vi "LJStreamUD.vi"() -> ()   [LabVIEW 2020]
uses:
  sub/LJstreamUD globals.vi
panel:
  out "Command Response  Error Message":string
  in  "Save Current Config":bool
  in  "Change Working Directory":bool
  in  "SettlingFactor":i32
  in  "Resolution":i32=1
  in  "Max File Size (Bytes)":i32=1048576 min=1 max=2000000000
  in  "Graph?":bool[](array[boolean])=[TRUE]
  out "Address":string
  in  "Disable Scaling*":bool=TRUE
  out "Device Type":string
  in  "stop stream":bool
  in  "exit":bool
  in  "# Scans On Graph":i32=1000 min=0
  out "Channel Config":T1={"# Channels"=4, "+Ch"=["0", "1", "2", "3", "4", "5", "6", "7"], "-Ch (U3)"=["31", "31", "31", "31", "31", "31", "31", "31"], "Ranges (UE9)"=[0, 0, 0, 0, 0, 0, 0, 0], "Scaling Equation"=["y=v0", "y=v1", "y=v2", "y=v3", "y=v4", "y=v5", "y=v6", "y=v7"]} {"Ranges (UE9)" items=["LJ_rgBIP5V", "LJ_rgUNI5V", "LJ_rgUNI2P5V", "LJ_rgUNI1P25V", "LJ_rgUNIP625V"]}
  out "Scaled":dbl[](array[numeric]) format="%.6f"
  in  "Scaling Equation":string[](array[string])=["y=a", "y=b", "y=c", "y=d", "y=e", "y=f", "y=g", "y=h", "y=i", "y=j", "y=k", "y=l", "y=m", "y=n", "y=o", "y=p"]
  in  "# Channels":i32=1 min=1
  in  "-Ch":string[](array[string])=["199", "199", "199", "199", "199", "199", "199", "199", "199", "199", "199", "199", "199", "199", "199", "199"]
  out "Voltage":dbl[](array[numeric]) format="%.6f"
  in  "Ranges":u16[](array[ring])=[0, 0, 0, 0, 0, 0, 0, 0, 0, 0, 0, 0, 0, 0, 0, 0] items=["LJ_rgBIP10V", "LJ_rgBIP5V", "LJ_rgUNI5V", "LJ_rgUNI2P5V", "LJ_rgUNI1P25V", "LJ_rgBIP1V", "LJ_rgUNIP625V", "LJ_rgBIPP1V", "LJ_rgBIPP01V"]
  out "?":cluster{dbl, dbl, dbl[][]}(graph)
  out "UD Backlog [%]":dbl format="%.2f"
  in  "+Ch":string[](array[string])=["0", "1", "2", "3", "4", "5", "6", "7", "8", "9", "10", "11", "12", "13", "14", "15"]
  out "ms Per Loop":u32
  out "Device Backlog [%]":dbl format="%.2f"
  out "# Scans Read":i32
  out "# of iterations":i32
  in  "Scan Rate (Hz)":dbl=500.0 format="%.3f"
  out "Current Data File":path
  in  "Data File Prefix":string="data"
  in  "Write To File":bool
  in  "start stream":bool caption="Start Stream"
  out "Last Stream Error Message":string
  # "0"
  # "1"
  # "2"
  # "3"
  # "4"
  # "5"
  # "6"
  # "7"
  # "8"
  # "9"
  # "10"
  # "11"
  # "12"
  # "13"
  # "14"
  # "15"
  # "*Scaling is computing intensive.  \nIf  the UD Backlog  is growing, disable scaling."
  # "# Iterations"
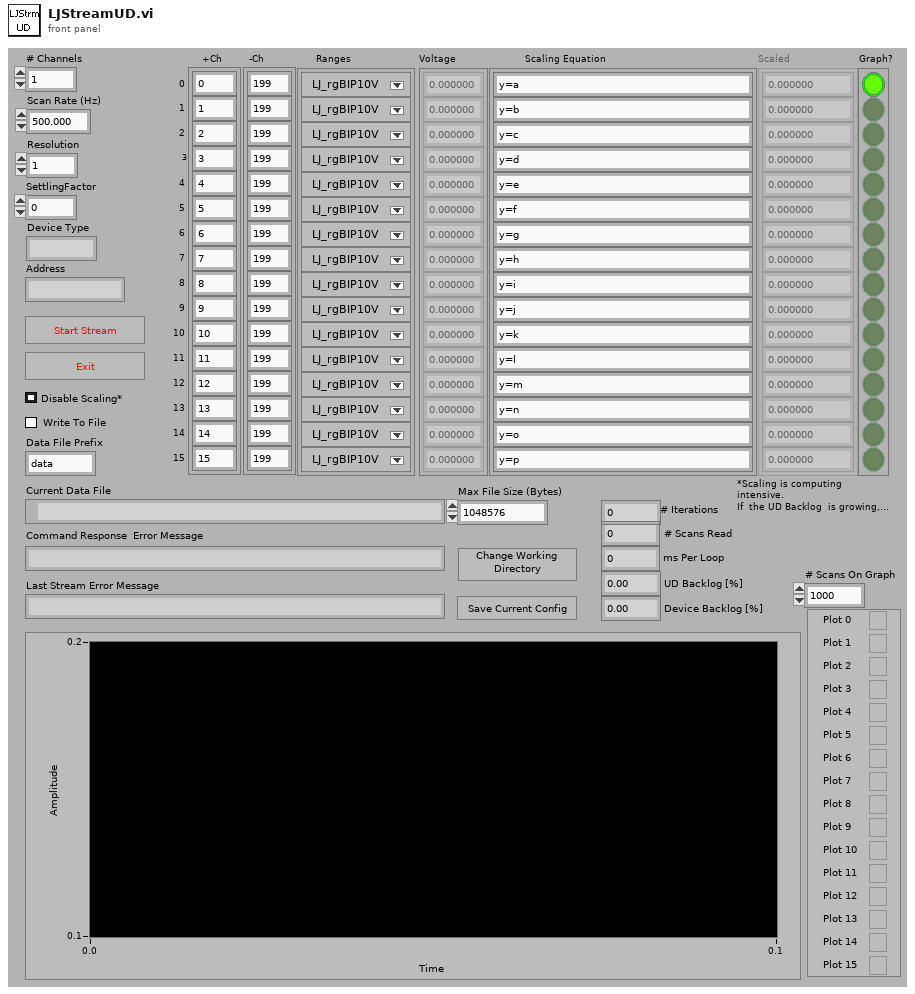
[diagram p1: front panel]
types:
  T1 = cluster{"# Channels":i32, "+Ch":string[], "-Ch (U3)":string[], "Ranges (UE9)":u16[], "Scaling Equation":string[]}
  T2 = cluster{"+Ch":string[], "-Ch":string[], "Ranges":u16[], "Scaling Equation":string[], "Graph?":bool[]}
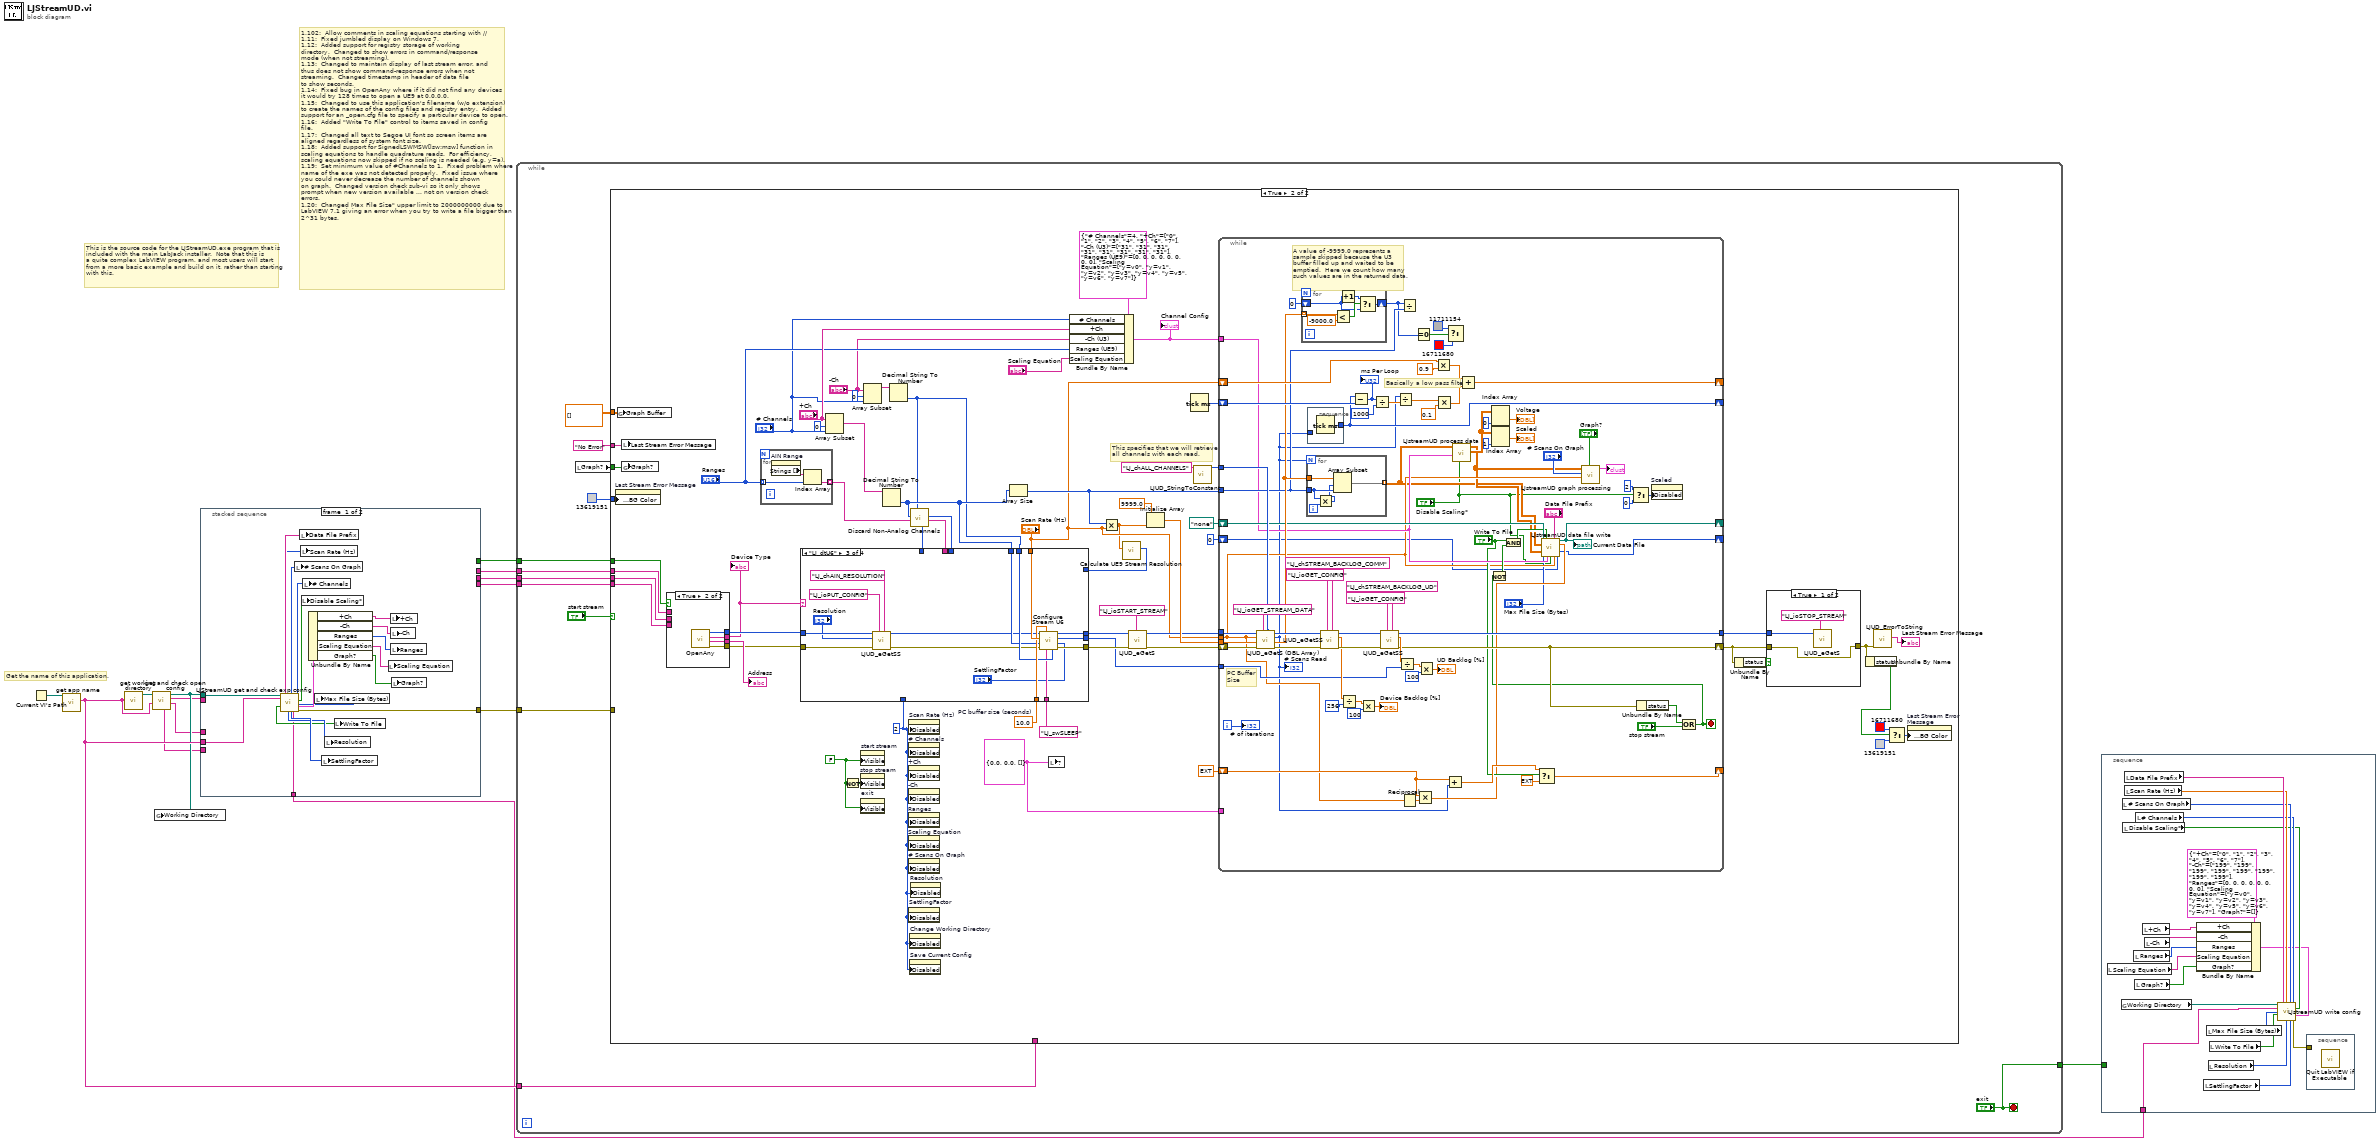
[diagram p0: block diagram]
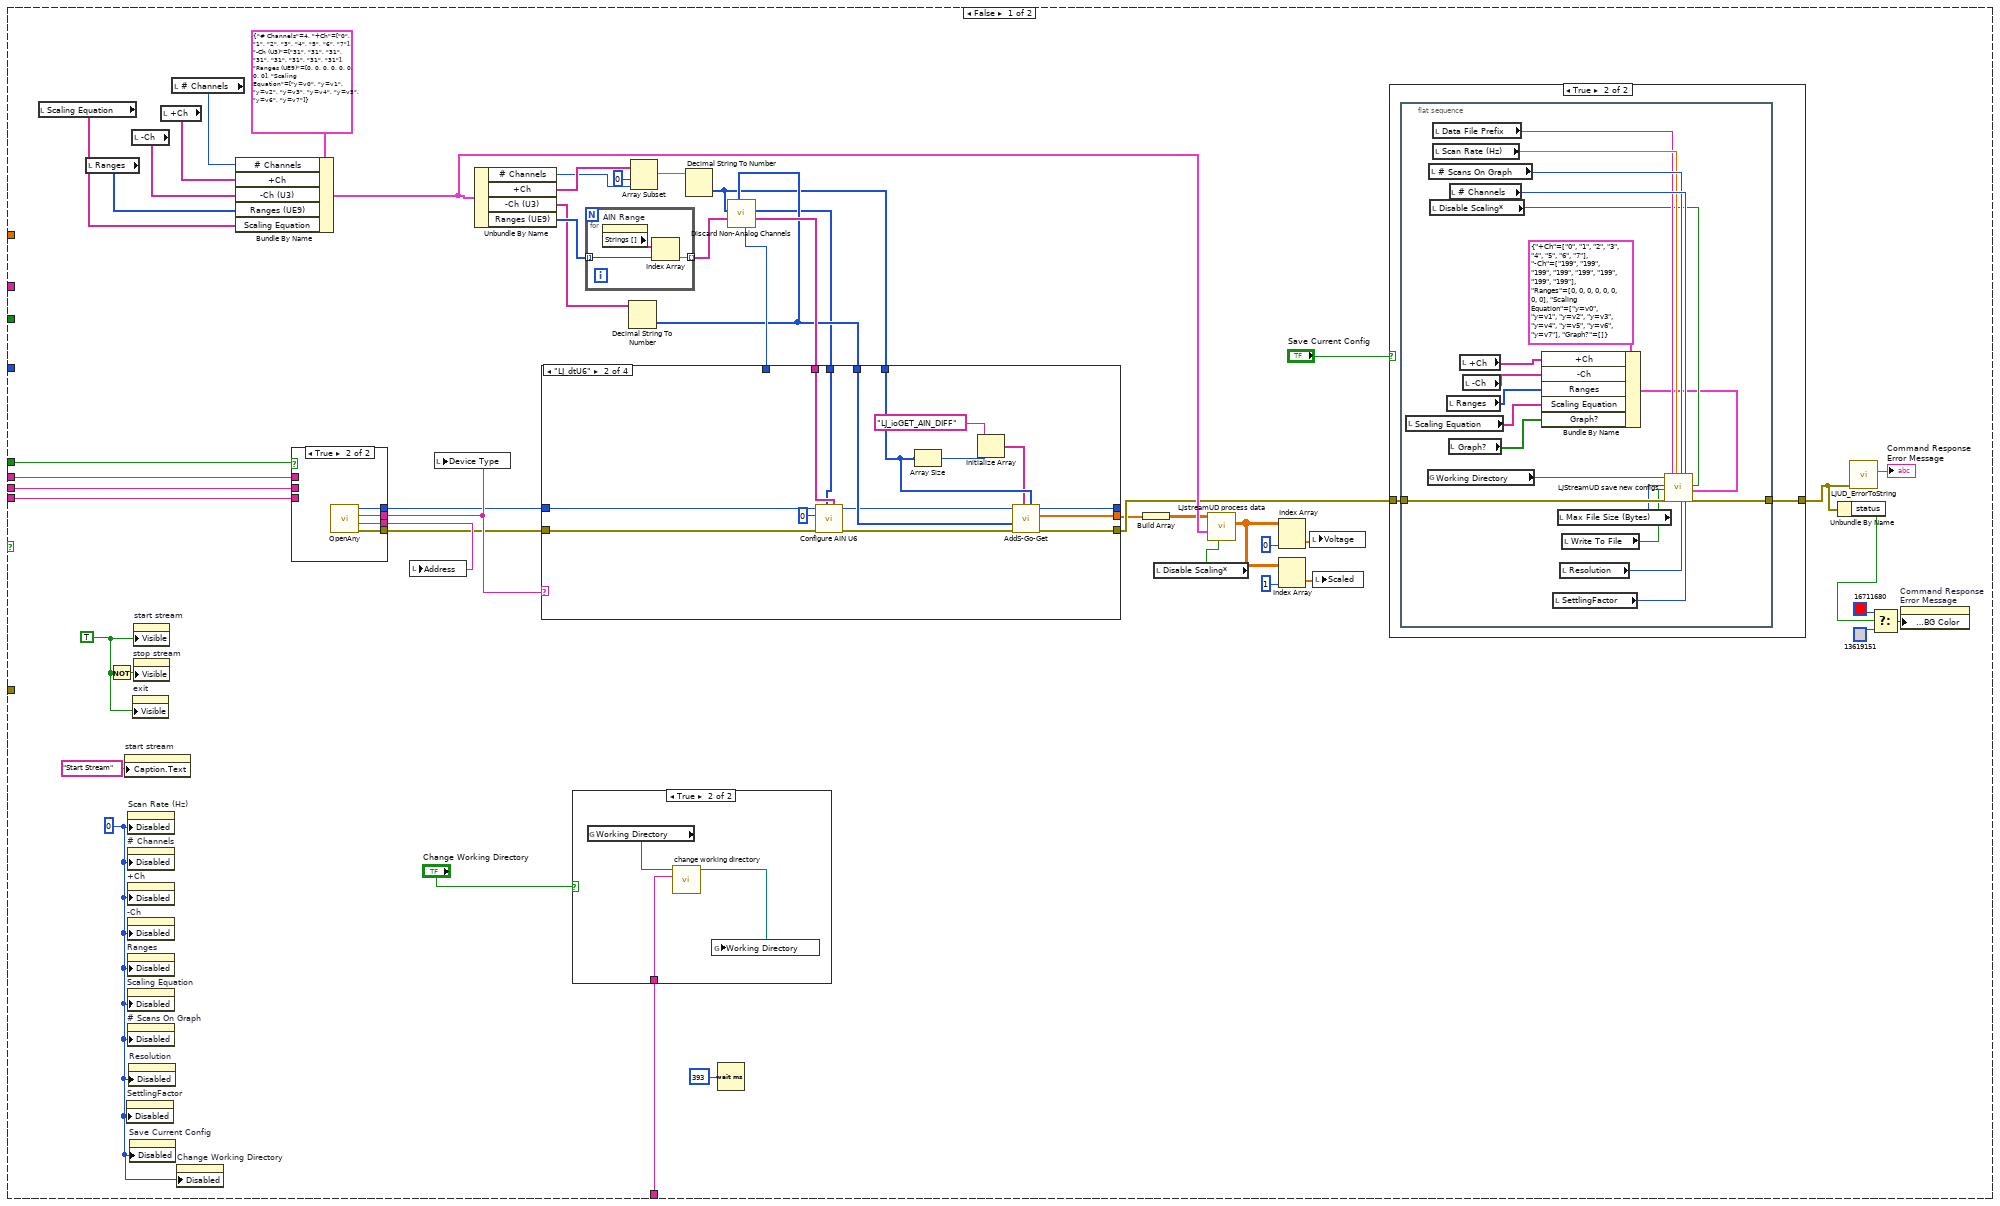
[diagram p2: hidden frame]
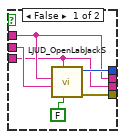
[diagram p4: hidden frame]
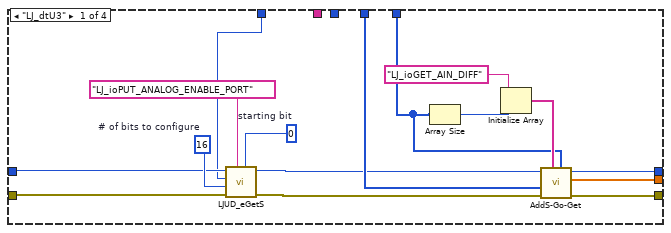
[diagram p6: hidden frame]
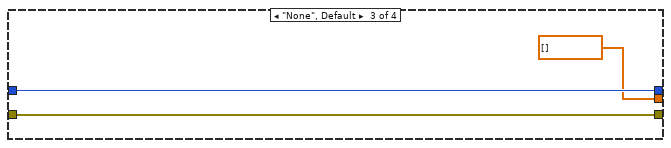
[diagram p7: hidden frame]
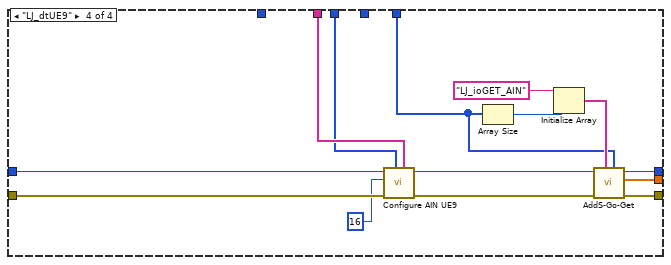
[diagram p8: hidden frame]
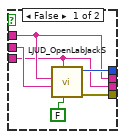
[diagram p9: hidden frame]
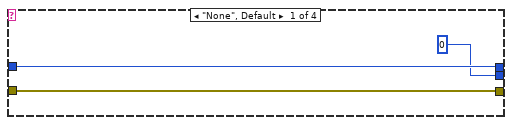
[diagram p10: hidden frame]
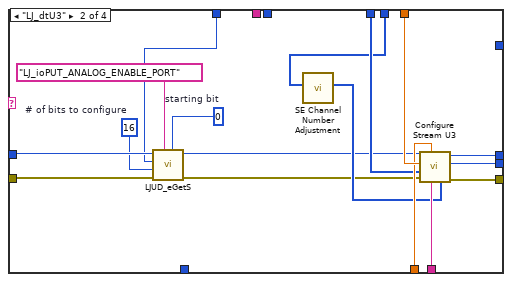
[diagram p11: hidden frame]
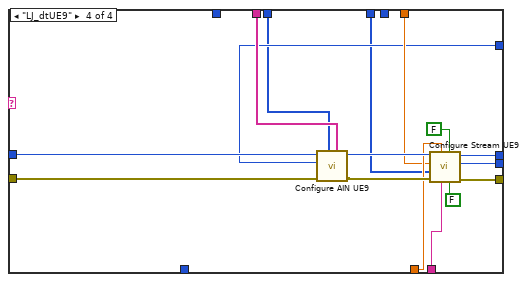
[diagram p12: hidden frame]
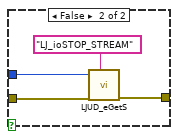
[diagram p13: hidden frame]
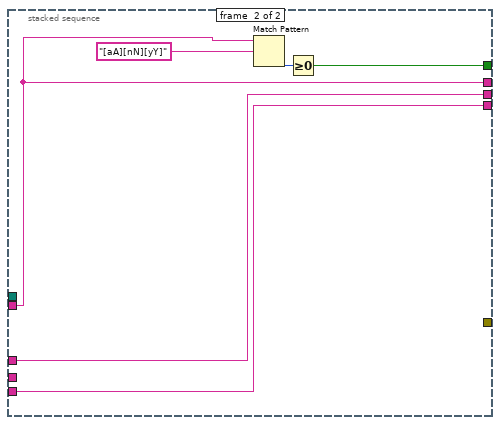
[diagram p14: hidden frame]
diagram:
  # "This is the source code for the LJStreamUD.exe program that is\nincluded with the main LabJack installer.  Note that this is \na quite complex LabVIEW program, and most users will start\nfrom a more basic example and build on it, rather than starting\nwith this."
  # "Get the name of this application."
  # "1.102:  Allow comments in scaling equations starting with //\n1.11:  Fixed jumbled display on Windows 7.\n1.12:  Added support for registry storage of working\ndirectory.  Changed to show errors in command/response\nmode (when not streaming).\n1.13:  Changed to maintain display of last stream error, and\nthus does not show command-response errors when not\nstreaming.  Changed timestamp in header of data file\nto show seconds.\n1.14:  Fixed bug in OpenAny where if it did not find any devices\nit would try 128 times to open a UE9 at 0.0.0.0.\n1.15:  Changed to use this application's filename (w/o extension)\nto create the names of the config files and registry entry.  Added\nsupport for an _open.cfg file to specify a particular device to open.\n1.16:  Added \"Write To File\" control to items saved in config\nfile.\n1.17:  Changed all text to Segoe UI font so screen items are\naligned regardless of system font size.\n1.18:  Added support for SignedLSWMSW[lsw:msw] function in\nscaling equations to handle quadrature reads.  For efficiency,\nscaling equations now skipped if no scaling is needed (e.g. y=a).\n1.19:  Set minimum value of #Channels to 1.  Fixed problem where\nname of the exe was not detected properly.  Fixed issue where\nyou could never decrease the number of channels shown\non graph.  Changed version check sub-vi so it only shows\nprompt when new version available ... not on version check\nerrors.\n1.20:  Changed Max File Size\" upper limit to 2000000000 due to\nLabVIEW 7.1 giving an error when you try to write a file bigger than\n2^31 bytes."
  n1 = Current VI's Path() -> (path=w9:path)
  n2 = call "get app name.vi"("Current VI's Path"=w9) -> ("App Name Without Extension"=w7:string)  [unwired: 4 in, 2 out]
  n3 = call "get working directory.vi"("Application Name"=w7) -> ("Working Directory"=w8:path)  [unwired: 9 in, 1 out]
  n4 = call "get and check open config.vi"("App Name"=w7, "Working Directory In"=w8) -> ("ConnectionType"=w4:string, "DeviceType"=w5:string, "Working Directory Out"=w6:path, "Identifier"=w3:string)  [unwired: 4 in, 2 out]
  n5 = global write "LJstreamUD globals.vi" "Working Directory"(w6) -> ()
  n6 = stacked-sequence {
    tunnel: w6 -> [w19 _]
    tunnel: w7 -> [w15 _]
    tunnel: [_ w37] -> w13
    tunnel: [_ w36] -> w12
    tunnel: [_ w35] -> w11
    tunnel: [_ w34] -> w10
    tunnel: w5 -> [_ w36]
    tunnel: w4 -> [_ w35]
    tunnel: w3 -> [_ w34]
    tunnel: [w17 _] -> w2
    tunnel: [w16 _] -> w1
    frame #0 {
      n7 = call "LJStreamUD get and check exp config.vi"("Working Directory In"=w19, "App Name"=w15) -> ("Write To File"=w18:bool, "Data File Prefix"=w27:string, "Interval (ms)"=w26:u32, "Resolution"=w20:u8, "Graph History"=w25:i32, "SettlingFactor"=w21:u8, "Device Config File Name"=w17:string, "# Channels"=w24:i32, "Disable Scaling"=w23:bool, "Max File Size (Bytes)"=w22:i32, "Channel Setup"=w33:T2, "error out"=w16:errorcluster)  [unwired: 6 in]
      n8 = local write "# Scans On Graph"(w25) -> ()
      n9 = local write "Data File Prefix"(w27) -> ()
      n10 = local write "Scan Rate (Hz)"(w26) -> ()
      n11 = local write "Disable Scaling*"(w23) -> ()
      n12 = local write "# Channels"(w24) -> ()
      n13 = Unbundle By Name(w33) -> ("+Ch"=w32:string[], "-Ch"=w31:string[], "Ranges"=w30:u16[], "Scaling Equation"=w29:string[], "Graph?"=w28:bool[])
      n14 = local write "Max File Size (Bytes)"(w22) -> ()
      n15 = local write "SettlingFactor"(w21) -> ()
      n16 = local write "Resolution"(w20) -> ()
      n17 = local write "Write To File"(w18) -> ()
      n18 = local write "Scaling Equation"(w29) -> ()
      n19 = local write "+Ch"(w32) -> ()
      n20 = local write "-Ch"(w31) -> ()
      n21 = local write "Ranges"(w30) -> ()
      n22 = local write "Graph?"(w28) -> ()
    }
    frame #1 {
      n23 = Match Pattern(string=w36, regular expression="[aA][nN][yY]") -> (offset past match=w38:i32)  [unwired: 1 in, 3 out]
      n24 = Greater Or Equal To 0?(x=w38) -> (x >= 0?=w37:bool)
    }
  }
  n25 = while {
    tunnel: w7 -> [w45]
    tunnel: ["exit"] -> w14
    tunnel: w13 -> [w44]
    tunnel: w12 -> [w43]
    tunnel: w11 -> [w42]
    tunnel: w10 -> [w41]
    tunnel: w1 -> [w40]
    stop <- "exit" stop-if-true
    n26 = local read "Graph?"() -> (w47:bool[])
    n27 = case shown="True" "start stream" {
      tunnel: "No Error" ("Error Message") -> [_ w215]
      tunnel: dbl[][] [] ("Graph Buffer") -> [_ w207]
      tunnel: w47 -> [_ w206]
      tunnel: u32 13619151 -> [_ w200]
      tunnel: w45 -> [w87 _]
      tunnel: w44 -> [w86 w195]
      tunnel: w43 -> [w85 w194]
      tunnel: w42 -> [w84 w193]
      tunnel: w41 -> [w83 w192]
      tunnel: w40 -> [_ _]
      frame False {
        w81 = TRUE ("Visible")
        w52 = u8 0 ("Disabled")
        n28 = local read "Scaling Equation"() -> (w56:string[])
        n29 = local read "Ranges"() -> (w57:u16[])
        n30 = Not(x=w81) -> (.not. x?=w100:bool)
        n31 = property on="start stream" class="Bool"("Caption.Text"="Start Stream") -> ()  [unwired: 2 in, 2 out]
        n32 = property on="SettlingFactor" class="DigNum (strict)"("Disabled"=w52) -> ()  [unwired: 2 in, 2 out]
        n33 = property on="Scan Rate (Hz)" class="DigNum (strict)"("Disabled"=w52) -> ()  [unwired: 2 in, 2 out]
        n34 = property on="# Channels" class="DigNum (strict)"("Disabled"=w52) -> ()  [unwired: 2 in, 2 out]
        n35 = property on="+Ch" class="Arr (strict)"("Disabled"=w52) -> ()  [unwired: 2 in, 2 out]
        n36 = property on="-Ch" class="Arr (strict)"("Disabled"=w52) -> ()  [unwired: 2 in, 2 out]
        n37 = property on="Ranges" class="Arr (strict)"("Disabled"=w52) -> ()  [unwired: 2 in, 2 out]
        n38 = property on="Scaling Equation" class="Arr (strict)"("Disabled"=w52) -> ()  [unwired: 2 in, 2 out]
        n39 = property on="# Scans On Graph" class="DigNum (strict)"("Disabled"=w52) -> ()  [unwired: 2 in, 2 out]
        n40 = property on="Resolution" class="DigNum (strict)"("Disabled"=w52) -> ()  [unwired: 2 in, 2 out]
        n41 = property on="Save Current Config" class="Bool"("Disabled"=w52) -> ()  [unwired: 2 in, 2 out]
        n42 = local read "-Ch"() -> (w58:string[])
        n43 = property on="exit" class="Bool"("Visible"=w81) -> ()  [unwired: 2 in, 2 out]
        n44 = property on="start stream" class="Bool"("Visible"=w81) -> ()  [unwired: 2 in, 2 out]
        n45 = property on="stop stream" class="Bool"("Visible"=w100) -> ()  [unwired: 2 in, 2 out]
        n46 = local read "+Ch"() -> (w59:string[])
        n47 = local read "# Channels"() -> (w60:i32)
        n48 = property on="Change Working Directory" class="Bool"("Disabled"=w52) -> ()  [unwired: 2 in, 2 out]
        n49 = Bundle By Name(cluster=T1 {"# Channels"=4, "+Ch"=["0", "1", "2", "3", "4", "5", "6", "7"], "-Ch (U3)"=["31", "31", "31", "31", "31", "31", "31", "31"], "Ranges (UE9)"=[0, 0, 0, 0, 0, 0, 0, 0], "Scaling Equation"=["y=v0", "y=v1", "y=v2", "y=v3", "y=v4", "y=v5", "y=v6", "y=v7"]} ("Channel Config"), "# Channels"=w60, "+Ch"=w59, "-Ch (U3)"=w58, "Ranges (UE9)"=w57, "Scaling Equation"=w56) -> (w93:T1)
        n50 = case shown="True" w86 {
          tunnel: [w129 w136] -> w95
          tunnel: [w127 w135] -> w94
          tunnel: [w132 w134] -> w92
          tunnel: [w131 w133] -> w91
          tunnel: w85 -> [w129 _]
          tunnel: w84 -> [w128 _]
          tunnel: w83 -> [w127 _]
          frame False {
            n51 = call "LJUD_OpenLabJackS.vi"("FirstFound"=FALSE, "Address"=w127, "ConnectionType"=w128, "DeviceType"=w129) -> ("error out"=w131:errorcluster, "Handle"=w132:i32)  [unwired: 5 in, 1 out]
          }
          frame True {
            n52 = call "OpenAny.vi"() -> ("error out"=w133:errorcluster, "Address Found"=w135:string, "Device Type Found"=w136:string, "Handle"=w134:i32)  [unwired: 8 in]
          }
        }
        n53 = local write "Address"(w94) -> ()
        n54 = local write "Device Type"(w95) -> ()
        n55 = Unbundle By Name(w93) -> ("# Channels"=w66:i32, "+Ch"=w67:string[], "-Ch (U3)"=w62:string[], "Ranges (UE9)"=w64:u16[])
        n56 = case shown="True" "Change Working Directory" {
          tunnel: w87 -> [_ w137]
          frame False {
          }
          frame True {
            n57 = global read "LJstreamUD globals.vi" "Working Directory"() -> (w139:path)
            n58 = call "change working directory.vi"("Application Name"=w137, "Working Directory In"=w139) -> ("Working Directory Out"=w138:path)  [unwired: 9 in]
            n59 = global write "LJstreamUD globals.vi" "Working Directory"(w138) -> ()
          }
        }
        n60 = for {
          tunnel: w64 -> [w103] mode=indexing
          tunnel: [w102] -> w63 mode=indexing
          n61 = property on="AIN Range" class="Ring (strict)"() -> ("Strings []"=w104:string[])  [unwired: 2 in, 2 out]
          n62 = Index Array(array=w104, index=w103) -> (element=w102:string)
        }
        n63 = Decimal String To Number(string=w62) -> (number=w96:i32[])  [unwired: 2 in, 1 out]
        n64 = Array Subset(array=w67, index=0 ("Array Index"), length=w66) -> (w65:string[])
        n65 = Decimal String To Number(string=w65) -> (number=w89:i32[])  [unwired: 2 in, 1 out]
        n66 = Wait (ms)(milliseconds to wait=u32 393) -> ()  [unwired: 1 out]
        n67 = call "Discard Non-Analog Channels.vi"("Channels In (-)"=w96, "Ranges In"=w63, "Channels In"=w89) -> ("Ranges Out"=w98:string[], "Channels Out"=w90:i32[], "FIO/EIO Analog Enable"=w97:i32)  [unwired: 5 in, 1 out]
        n68 = case shown="\"LJ_dtU6\"" w95 {
          tunnel: w97 -> [w141 _ _ _]
          tunnel: w91 -> [w145 w164 w172 w186]
          tunnel: w92 -> [w144 w165 w173 w187]
          tunnel: w98 -> [_ w166 _ w185]
          tunnel: w90 -> [_ w163 _ w175]
          tunnel: [w151 w169 w173 w178] -> _
          tunnel: [w152 w170 w172 w177] -> w76
          tunnel: [w150 w168 dbl[] [] ("Values Read") w176] -> w54
          tunnel: w96 -> [w149 w167 _ _]
          tunnel: w89 -> [w140 w162 _ w174]
          frame "LJ_dtU3" {
            w148 = 0  # starting bit
            w146 = 16  # # of bits to configure
            n69 = call "LJUD_eGetS.vi"("Channel"=w148, "IOType"="LJ_ioPUT_ANALOG_ENABLE_PORT" ("Channel"), "error in"=w145, "x1"=w146, "Value Write"=w141, "Handle In"=w144) -> ("error out"=w143:errorcluster, "Handle Out"=w142:i32)  [unwired: 3 in, 1 out]
            n70 = Array Size(array=w140) -> (size(s)=w154:i32)
            n71 = Initialize Array("LJ_ioGET_AIN_DIFF" ("IOType"), w154) -> (w155:string[])
            n72 = call "AddS-Go-Get.vi"("Channels"=w140, "IOTypes"=w155, "error in"=w143, "x1"=w149, "Handle In"=w142) -> ("error out"=w152:errorcluster, "Values Read"=w150:dbl[], "Handle Out"=w151:i32)  [unwired: 4 in]
          }
          frame "LJ_dtU6" {
            n73 = call "Configure AIN U6.vi"("Ranges"=w166, "Positive Channels"=w163, "error in"=w164, "Resolution"=0, "Handle In"=w165) -> ("error out"=w158:errorcluster, "Handle Out"=w157:i32)  [unwired: 5 in]
            n74 = Array Size(array=w162) -> (size(s)=w160:i32)
            n75 = Initialize Array("LJ_ioGET_AIN_DIFF" ("IOType"), w160) -> (w161:string[])
            n76 = call "AddS-Go-Get.vi"("Channels"=w162, "IOTypes"=w161, "error in"=w158, "x1"=w167, "Handle In"=w157) -> ("error out"=w170:errorcluster, "Values Read"=w168:dbl[], "Handle Out"=w169:i32)  [unwired: 4 in]
          }
          frame "None", Default {
          }
          frame "LJ_dtUE9" {
            n77 = call "Configure AIN UE9.vi"("Ranges"=w185, "Channels"=w175, "error in"=w186, "Resolution"=16, "Handle In"=w187) -> ("error out"=w179:errorcluster, "Handle Out"=w180:i32)  [unwired: 5 in]
            n78 = Array Size(array=w174) -> (size(s)=w182:i32)
            n79 = Initialize Array("LJ_ioGET_AIN" ("IOType"), w182) -> (w183:string[])
            n80 = call "AddS-Go-Get.vi"("Channels"=w174, "IOTypes"=w183, "error in"=w179, "Handle In"=w180) -> ("error out"=w177:errorcluster, "Values Read"=w176:dbl[], "Handle Out"=w178:i32)  [unwired: 5 in]
          }
        }
        n81 = Build Array(w54) -> (w75:dbl[][])
        n82 = local read "Disable Scaling*"() -> (w69:bool)
        n83 = call "LJstreamUD process data.vi"("Disable Scaling"=w69, "Channel Config"=w93, "Voltages"=w75) -> ("Volts,Scaled Averages"=w72:dbl[][])  [unwired: 7 in, 1 out]
        n84 = Index Array(array=w72, index (col)=0 ("Disabled Index (col)")) -> (element=w71:dbl[])  [unwired: 1 in]
        n85 = Index Array(array=w72, index (col)=1 ("Disabled Index (col)")) -> (element=w70:dbl[])  [unwired: 1 in]
        n86 = local write "Voltage"(w71) -> ()
        n87 = local write "Scaled"(w70) -> ()
        n88 = case shown="True" "Save Current Config" {
          tunnel: w76 -> [w105 w107]
          tunnel: [w105 w106] -> w77
          frame False {
          }
          frame True {
            n89 = flat-sequence {
              tunnel: w107 -> [w126]
              tunnel: [w125] -> w106
              frame #0 {
                n90 = local read "Scaling Equation"() -> (w118:string[])
                n91 = global read "LJstreamUD globals.vi" "Working Directory"() -> (w123:path)
                n92 = local read "# Scans On Graph"() -> (w112:i32)
                n93 = local read "Disable Scaling*"() -> (w109:bool)
                n94 = local read "Data File Prefix"() -> (w110:string)
                n95 = local read "Scan Rate (Hz)"() -> (w111:dbl)
                n96 = local read "Ranges"() -> (w117:u16[])
                n97 = local read "Graph?"() -> (w119:bool[])
                n98 = local read "# Channels"() -> (w113:i32)
                n99 = local read "+Ch"() -> (w115:string[])
                n100 = local read "-Ch"() -> (w116:string[])
                n101 = Bundle By Name(cluster=T2 {"+Ch"=["0", "1", "2", "3", "4", "5", "6", "7"], "-Ch"=["199", "199", "199", "199", "199", "199", "199", "199"], "Ranges"=[0, 0, 0, 0, 0, 0, 0, 0], "Scaling Equation"=["y=v0", "y=v1", "y=v2", "y=v3", "y=v4", "y=v5", "y=v6", "y=v7"], "Graph?"=[]} ("Channel Setup"), "+Ch"=w115, "-Ch"=w116, "Ranges"=w117, "Scaling Equation"=w118, "Graph?"=w119) -> (w108:T2)
                n102 = local read "SettlingFactor"() -> (w121:i32)
                n103 = local read "Max File Size (Bytes)"() -> (w120:i32)
                n104 = local read "Resolution"() -> (w122:i32)
                n105 = local read "Write To File"() -> (w124:bool)
                n106 = call "LJStreamUD save new configs.vi"("Working Directory"=w123, "Max File Size (Bytes)"=w120, "Write To File"=w124, "error in"=w126, "Data File Prefix"=w110, "Scan Rate (Hz)"=w111, "Graph History"=w112, "Resolution"=w122, "# Channels"=w113, "SettlingFactor"=w121, "Disable Scaling"=w109, "Channel Setup"=w108) -> ("error out"=w125:errorcluster)  [unwired: 6 in, 1 out]
              }
            }
          }
        }
        n107 = Unbundle By Name(w77) -> ("status"=w55:bool)
        n108 = call "LJUD_ErrorToString.vi"("error in"=w77) -> ("String"=→"Command Response  Error Message":string)  [unwired: 10 in]
        n109 = Select(t=u32 16711680, s=w55, f=u32 13619151) -> (s? t:f=w78:u32)
        n110 = property on="Command Response  Error Message" class="Str"("Text.Text Colors:BG Color"=w78) -> ()  [unwired: 2 in, 2 out]
      }
      frame True {
        w190 = FALSE ("Visible")
        w188 = u8 2 ("Disabled")
        w217 = cluster{dbl, dbl, dbl[][]} {0.0, 0.0, []} ("Waveform Graph")
        w234 = 10.0  # PC buffer size (seconds)
        # "This specifies that we will retrieve\nall channels with each read."
        n111 = property on="Last Stream Error Message" class="Str"("Text.Text Colors:BG Color"=w200) -> ()  [unwired: 2 in, 2 out]
        n112 = global write "LJstreamUD globals.vi" "Graph Buffer"(w207) -> ()
        n113 = local write "Last Stream Error Message"(w215) -> ()
        n114 = global write "LJstreamUD globals.vi" "Graph?"(w206) -> ()
        n115 = case shown="True" w195 {
          tunnel: [w252 w259] -> w198
          tunnel: [w250 w258] -> w197
          tunnel: [w255 w257] -> w199
          tunnel: [w254 w256] -> w196
          tunnel: w194 -> [w252 _]
          tunnel: w193 -> [w251 _]
          tunnel: w192 -> [w250 _]
          frame False {
            n116 = call "LJUD_OpenLabJackS.vi"("FirstFound"=FALSE, "Address"=w250, "ConnectionType"=w251, "DeviceType"=w252) -> ("error out"=w254:errorcluster, "Handle"=w255:i32)  [unwired: 5 in, 1 out]
          }
          frame True {
            n117 = call "OpenAny.vi"() -> ("error out"=w256:errorcluster, "Address Found"=w258:string, "Device Type Found"=w259:string, "Handle"=w257:i32)  [unwired: 8 in]
          }
        }
        "Device Type" <- w198
        "Address" <- w197
        n118 = for {
          tunnel: "Ranges" -> [w353] mode=indexing
          tunnel: [w352] -> w229 mode=indexing
          n119 = property on="AIN Range" class="Ring (strict)"() -> ("Strings []"=w354:string[])  [unwired: 2 in, 2 out]
          n120 = Index Array(array=w354, index=w353) -> (element=w352:string)
        }
        n121 = Array Subset(array="+Ch", index=0 ("Array Index"), length="# Channels") -> (w226:string[])
        n122 = Not(x=w190) -> (.not. x?=w216:bool)
        n123 = property on="start stream" class="Bool"("Visible"=w190) -> ()  [unwired: 2 in, 2 out]
        n124 = property on="stop stream" class="Bool"("Visible"=w216) -> ()  [unwired: 2 in, 2 out]
        n125 = property on="exit" class="Bool"("Visible"=w190) -> ()  [unwired: 2 in, 2 out]
        n126 = Array Subset(array="-Ch", index=0 ("Array Index"), length="# Channels") -> (w210:string[])
        n127 = Decimal String To Number(string=w226) -> (number=w214:i32[])  [unwired: 2 in, 1 out]
        n128 = Decimal String To Number(string=w210) -> (number=w212:i32[])  [unwired: 2 in, 1 out]
        n129 = property on="Scan Rate (Hz)" class="DigNum (strict)"("Disabled"=w188) -> ()  [unwired: 2 in, 2 out]
        n130 = property on="# Channels" class="DigNum (strict)"("Disabled"=w188) -> ()  [unwired: 2 in, 2 out]
        n131 = property on="+Ch" class="Arr (strict)"("Disabled"=w188) -> ()  [unwired: 2 in, 2 out]
        n132 = property on="-Ch" class="Arr (strict)"("Disabled"=w188) -> ()  [unwired: 2 in, 2 out]
        n133 = property on="Ranges" class="Arr (strict)"("Disabled"=w188) -> ()  [unwired: 2 in, 2 out]
        n134 = property on="Scaling Equation" class="Arr (strict)"("Disabled"=w188) -> ()  [unwired: 2 in, 2 out]
        n135 = property on="# Scans On Graph" class="DigNum (strict)"("Disabled"=w188) -> ()  [unwired: 2 in, 2 out]
        n136 = property on="SettlingFactor" class="DigNum (strict)"("Disabled"=w188) -> ()  [unwired: 2 in, 2 out]
        n137 = property on="Change Working Directory" class="Bool"("Disabled"=w188) -> ()  [unwired: 2 in, 2 out]
        n138 = property on="Save Current Config" class="Bool"("Disabled"=w188) -> ()  [unwired: 2 in, 2 out]
        n139 = call "Discard Non-Analog Channels.vi"("Channels In (-)"=w212, "Ranges In"=w229, "Channels In"=w214) -> ("Ranges Out"=w228:string[], "Channels Out"=w213:i32[], "FIO/EIO Analog Enable"=w235:i32)  [unwired: 5 in, 1 out]
        n140 = property on="Resolution" class="DigNum (strict)"("Disabled"=w188) -> ()  [unwired: 2 in, 2 out]
        n141 = Array Size(array=w214) -> (size(s)=w246:i32)
        n142 = local write item#12(w217) -> ()
        n143 = Bundle By Name(cluster=T1 {"# Channels"=4, "+Ch"=["0", "1", "2", "3", "4", "5", "6", "7"], "-Ch (U3)"=["31", "31", "31", "31", "31", "31", "31", "31"], "Ranges (UE9)"=[0, 0, 0, 0, 0, 0, 0, 0], "Scaling Equation"=["y=v0", "y=v1", "y=v2", "y=v3", "y=v4", "y=v5", "y=v6", "y=v7"]} ("Channel Config"), "# Channels"="# Channels", "+Ch"="+Ch", "-Ch (U3)"="-Ch", "Ranges (UE9)"="Ranges", "Scaling Equation"="Scaling Equation") -> (w222:T1)
        "Channel Config" <- w222
        n144 = Multiply(x=w246, y="Scan Rate (Hz)") -> (x*y=w225:dbl)
        n145 = call "Calculate UE9 Stream Resolution.vi"("Sample Rate"=w225) -> ("Resolution"=w224:i32)  [unwired: 10 in]
        n146 = case shown="\"LJ_dtU6\"" w198 {
          tunnel: "Scan Rate (Hz)" -> [_ w374 w390 w395]
          tunnel: w235 -> [_ w359 _ _]
          tunnel: w196 -> [w357 w364 w381 w399]
          tunnel: w199 -> [w356 w362 w382 w400]
          tunnel: w234 -> [_ w373 w389 w398]
          tunnel: w212 -> [_ w366 w388 _]
          tunnel: w214 -> [_ w372 w387 w392]
          tunnel: [w357 w371 w386 w401] -> w233
          tunnel: [w356 w370 w385 w402] -> w232
          tunnel: [0 ("PC buffer size (samples)") w369 w384 w396] -> w231
          tunnel: "LJ_swSLEEP" ("Wait Mode (2)") -> [_ w368 w383 w397]
          tunnel: w228 -> [_ _ _ w394]
          tunnel: w224 -> [_ _ _ w393]
          tunnel: w188 -> [_ _ _ _]
          tunnel: w213 -> [_ _ _ w391]
          frame "None", Default {
          }
          frame "LJ_dtU3" {
            w358 = 16  # # of bits to configure
            w360 = 0  # starting bit
            n147 = call "LJUD_eGetS.vi"("Channel"=w360, "IOType"="LJ_ioPUT_ANALOG_ENABLE_PORT" ("Channel"), "error in"=w364, "x1"=w358, "Value Write"=w359, "Handle In"=w362) -> ("error out"=w363:errorcluster, "Handle Out"=w361:i32)  [unwired: 3 in, 1 out]
            n148 = call "SE Channel Number Adjustment.vi"("Channels In"=w366) -> ("Channels Out"=w367:i32[])  [unwired: 10 in]
            n149 = call "Configure Stream U3.vi"("Scan List (-)"=w367, "Wait Mode"=w368, "PC buffer size (seconds)"=w373, "error in"=w363, "Scan List (+)"=w372, "Scan Rate (Hz)"=w374, "Handle In"=w361) -> ("error out"=w371:errorcluster, "PC buffer size (samples)"=w369:i32, "Handle Out"=w370:i32)  [unwired: 2 in]
          }
          frame "LJ_dtU6" {
            n150 = call "LJUD_eGetSS.vi"("Channel"="LJ_chAIN_RESOLUTION" ("IOType"), "IOType"="LJ_ioPUT_CONFIG", "error in"=w381, "Value Write"="Resolution", "Handle In"=w382) -> ("error out"=w379:errorcluster, "Handle Out"=w380:i32)  [unwired: 4 in, 1 out]
            n151 = call "Configure Stream U6.vi"("SettlingFactor"="SettlingFactor", "Scan List (-)"=w388, "Wait Mode"=w383, "PC buffer size (seconds)"=w389, "error in"=w379, "Scan List (+)"=w387, "Scan Rate (Hz)"=w390, "Handle In"=w380) -> ("error out"=w386:errorcluster, "PC buffer size (samples)"=w384:i32, "Handle Out"=w385:i32)  [unwired: 1 in]
          }
          frame "LJ_dtUE9" {
            n152 = call "Configure AIN UE9.vi"("Ranges"=w394, "Channels"=w391, "error in"=w399, "Resolution"=w393, "Handle In"=w400) -> ("error out"=w404:errorcluster, "Handle Out"=w403:i32)  [unwired: 5 in]
            n153 = call "Configure Stream UE9.vi"("External Scan Trigger"=FALSE, "Scan Clock Output"=FALSE, "Wait Mode"=w397, "PC buffer size (seconds)"=w398, "error in"=w404, "Scan List"=w392, "Scan Rate (Hz)"=w395, "Handle In"=w403) -> ("error out"=w401:errorcluster, "PC buffer size (samples)"=w396:i32, "Handle Out"=w402:i32)  [unwired: 1 in]
          }
        }
        n154 = call "LJUD_eGetS.vi"("IOType"="LJ_ioSTART_STREAM", "error in"=w233, "Handle In"=w232) -> ("error out"=w237:errorcluster, "Handle Out"=w242:i32)  [unwired: 6 in, 1 out]
        n155 = Initialize Array(9999.0, w225) -> (w247:dbl[])
        n156 = Tick Count (ms)() -> (millisecond timer value=w243:u32)
        n157 = call "LJUD_StringToConstant.vi"("String"="LJ_chALL_CHANNELS") -> ("Constant Number"=w238:i32)  [unwired: 9 in, 1 out]
        n158 = while {
          shift-left: u32 0 ("Data File #") -> [w261]
          shift-right: [w262] -> _
          tunnel: w217 -> [_]
          shift-left: ext 0.0 -> [w278]
          shift-right: [w279] -> _
          tunnel: w222 -> [w283]
          tunnel: w231 -> [w304]
          shift-left: w237 -> [w312]
          shift-right: [w293] -> w236
          tunnel: w238 -> [w317]
          shift-left: "Scan Rate (Hz)" -> [w325]
          shift-right: [w322] -> _
          shift-left: w243 -> [w333]
          shift-right: [w330] -> _
          tunnel: [w294] -> w244
          tunnel: w246 -> [w299]
          tunnel: w247 -> [w335]
          tunnel: "Scan Rate (Hz)" -> [w276]
          shift-left: path "none" ("Current Data File Out") -> [w291]
          shift-right: [w292] -> _
          tunnel: w242 -> [w337]
          i -> [w334]
          stop <- w271 stop-if-true
          # "PC Buffer\nSize"
          # "A value of -9999.0 represents a\nsample skipped because the U3\nbuffer filled up and waited to be\nemptied.  Here we count how many\nsuch values are in the returned data."
          # "Basically a low pass filter"
          n159 = call "LJUD_eGetS (DBL Array).vi"("Channel"=w317, "IOType"="LJ_ioGET_STREAM_DATA", "error in"=w312, "DBL Array Write"=w335, "Value"=w276, "Handle In"=w337) -> ("error out"=w320:errorcluster, "DBL Array Read"=w301:dbl[], "Value"=w274:i32, "Handle Out"=w321:i32)  [unwired: 2 in]
          "# Scans Read" <- w274
          n160 = for {
            shift-right: [w340] -> w296
            shift-left: 0 -> [w341]
            tunnel: w301 -> [w344] mode=indexing
            n161 = Less?(x=w344, y=-9000.0) -> (x < y?=w342:bool)
            n162 = Increment(x=w341) -> (x+1=w345:i32)
            n163 = Select(t=w345, s=w342, f=w341) -> (s? t:f=w340:i32)
          }
          n164 = for {
            N: w274 -> [_]
            tunnel: w301 -> [w351]
            tunnel: w299 -> [w350]
            tunnel: [w347] -> w268 mode=indexing
            i -> [w349]
            n165 = Multiply(x=w350, y=w349) -> (x*y=w348:i32)
            n166 = Array Subset(array=w351, index=w348, length=w350) -> (w347:dbl[])
          }
          n167 = stacked-sequence {
            tunnel: w274 -> [_]
            tunnel: [w346] -> w330
            frame #0 {
              n168 = Tick Count (ms)() -> (millisecond timer value=w346:u32)
            }
          }
          n169 = call "LJUD_eGetSS.vi"("Channel"="LJ_chSTREAM_BACKLOG_COMM", "IOType"="LJ_ioGET_CONFIG", "error in"=w320, "Handle In"=w321) -> ("error out"=w313:errorcluster, "Value Read"=w308:dbl, "Handle Out"=w314:i32)  [unwired: 5 in]
          n170 = Divide(x=w308, y=256) -> (x/y=w311:dbl)
          n171 = Subtract(x=w330, y=w333) -> (x-y=w332:u32)
          "ms Per Loop" <- w332
          n172 = Multiply(x=w311, y=100) -> (x*y=→"Device Backlog [%]":dbl)
          n173 = Divide(x=w332, y=u32 1000) -> (x/y=w329:dbl)
          n174 = call "LJUD_eGetSS.vi"("Channel"="LJ_chSTREAM_BACKLOG_UD", "IOType"="LJ_ioGET_CONFIG", "error in"=w313, "Handle In"=w314) -> ("error out"=w293:errorcluster, "Value Read"=w303:dbl, "Handle Out"=w294:i32)  [unwired: 5 in]
          n175 = Divide(x=w274, y=w329) -> (x/y=w328:dbl)
          n176 = Divide(x=w303, y=w304) -> (x/y=w305:dbl)
          n177 = Divide(x=w296, y=w299) -> ()  [unwired: 1 out]
          n178 = Reciprocal(x=w276) -> (1/x=w282:dbl)
          n179 = Equal To 0?(x=w296) -> (x = 0?=w295:bool)
          n180 = Multiply(x=w278, y=w282) -> (x*y=w275:ext)
          n181 = Multiply(x=w305, y=100) -> (x*y=→"UD Backlog [%]":dbl)
          n182 = Multiply(x=w325, y=0.9) -> (x*y=w324:dbl)
          n183 = Multiply(x=w328, y=0.1) -> (x*y=w323:dbl)
          n184 = Add(x=w278, y=w274) -> (x+y=w280:ext)
          n185 = Select(t=u32 11711154, s=w295, f=u32 16711680) -> ()  [unwired: 1 out]
          n186 = call "LJstreamUD process data.vi"("Disable Scaling"="Disable Scaling*", "Channel Config"=w283, "Voltages"=w268) -> ("Volts,Scaled Averages"=w270:dbl[][], "Scaled Data"=w269:dbl[][])  [unwired: 7 in]
          n187 = Add(x=w324, y=w323) -> (x+y=w322:dbl)
          n188 = Index Array(array=w270, index (col)=0 ("Disabled Index (col)")) -> (element=→"Voltage":dbl[])  [unwired: 1 in]
          n189 = Index Array(array=w270, index (col)=1 ("Disabled Index (col)")) -> (element=→"Scaled":dbl[])  [unwired: 1 in]
          n190 = Select(t=w280, s="Write To File", f=ext 0.0) -> (s? t:f=w279:ext)
          n191 = call "LJstreamUD graph processing.vi"("Graph?"="Graph?", "Scan Rate"=w276, "Graph History (# scans)"="# Scans On Graph", "Scaled Data"=w269) -> ("Graph Data"=→"?":cluster{dbl, dbl, dbl[][]})  [unwired: 7 in]
          n192 = Select(t=u8 2, s="Disable Scaling*", f=u8 0) -> (s? t:f=w266:u8)
          n193 = Unbundle By Name(w293) -> ("status"=w272:bool)
          n194 = property on="Scaled" class="Arr (strict)"("Disabled"=w266) -> ()  [unwired: 2 in, 2 out]
          n195 = Compound Arithmetic op=OR(w272, "stop stream") -> (w271:bool)
          n196 = Not(x=w271) -> (.not. x?=w338:bool)
          n197 = And(x="Write To File", y=w338) -> (x .and. y?=w290:bool)
          n198 = call "LJstreamUD data file write.vi"("Current Data File In"=w291, "Write To File"=w290, "Data File Prefix"="Data File Prefix", "Voltages"=w268, "Time"=w275, "Scaled Data"=w269, "max file size (bytes)"="Max File Size (Bytes)", "Channel Config"=w283, "Disable Scaling"="Disable Scaling*", "Scan Rate"=w276, "Starting #"=w261) -> ("Current Data File Out"=w292:path, "Data File #"=w262:u32)  [unwired: 3 in]
          "Current Data File" <- w292
          "# of iterations" <- w334
        }
        n199 = Unbundle By Name(w236) -> ("status"=w240:bool)
        n200 = case shown="True" w240 {
          tunnel: w244 -> [w408 w412]
          tunnel: [w407 w411] -> w202
          tunnel: w236 -> [w407 w410]
          frame True {
            n201 = call "LJUD_eGetS.vi"("IOType"="LJ_ioSTOP_STREAM", "Handle In"=w408) -> ()  [unwired: 7 in, 3 out]
          }
          frame False {
            n202 = call "LJUD_eGetS.vi"("IOType"="LJ_ioSTOP_STREAM", "error in"=w410, "Handle In"=w412) -> ("error out"=w411:errorcluster)  [unwired: 6 in, 2 out]
          }
        }
        n203 = Unbundle By Name(w202) -> ("status"=w189:bool)
        n204 = call "LJUD_ErrorToString.vi"("error in"=w202) -> ("String"=→"Last Stream Error Message":string)  [unwired: 10 in]
        n205 = Select(t=u32 16711680, s=w189, f=u32 13619151) -> (s? t:f=w201:u32)
        n206 = property on="Last Stream Error Message" class="Str"("Text.Text Colors:BG Color"=w201) -> ()  [unwired: 2 in, 2 out]
      }
    }
  }
  n207 = stacked-sequence {
    tunnel: w14 -> [_]
    tunnel: w2 -> [w415]
    frame #0 {
      n208 = local read "Scaling Equation"() -> (w422:string[])
      n209 = global read "LJstreamUD globals.vi" "Working Directory"() -> (w416:path)
      n210 = local read "# Scans On Graph"() -> (w429:i32)
      n211 = local read "Disable Scaling*"() -> (w427:bool)
      n212 = local read "Data File Prefix"() -> (w431:string)
      n213 = local read "Scan Rate (Hz)"() -> (w430:dbl)
      n214 = local read "Ranges"() -> (w423:u16[])
      n215 = local read "Graph?"() -> (w421:bool[])
      n216 = local read "# Channels"() -> (w428:i32)
      n217 = local read "+Ch"() -> (w425:string[])
      n218 = local read "-Ch"() -> (w424:string[])
      n219 = Bundle By Name(cluster=T2 {"+Ch"=["0", "1", "2", "3", "4", "5", "6", "7"], "-Ch"=["199", "199", "199", "199", "199", "199", "199", "199"], "Ranges"=[0, 0, 0, 0, 0, 0, 0, 0], "Scaling Equation"=["y=v0", "y=v1", "y=v2", "y=v3", "y=v4", "y=v5", "y=v6", "y=v7"], "Graph?"=[]} ("Channel Setup"), "+Ch"=w425, "-Ch"=w424, "Ranges"=w423, "Scaling Equation"=w422, "Graph?"=w421) -> (w420:T2)
      n220 = local read "SettlingFactor"() -> (w418:i32)
      n221 = local read "Max File Size (Bytes)"() -> (w419:i32)
      n222 = local read "Resolution"() -> (w417:i32)
      n223 = local read "Write To File"() -> (w414:bool)
      n224 = call "LJstreamUD write config.vi"("Working Directory"=w416, "Data File Prefix"=w431, "Scan Rate (Hz)"=w430, "Graph History"=w429, "# Channels"=w428, "filename"=w415, "Disable Scaling"=w427, "Max File Size (Bytes)"=w419, "Write To File"=w414, "Channel Setup"=w420, "Resolution"=w417, "SettlingFactor"=w418) -> ("error out"=w432:errorcluster)  [unwired: 3 in]
      n225 = stacked-sequence {
        tunnel: w432 -> [_]
        frame #0 {
          n226 = call "Quit LabVIEW if Executable.vi"() -> ()  [unwired: 1 in]
        }
      }
    }
  }
